vi "Destroy.vi"(11 "Data Value Reference in":refnum<data-value>) -> ()   [LabVIEW 2021, in "d20.lvlib" / "Node.lvclass"]
uses:
  Node.lvclass
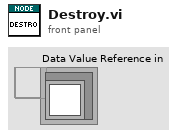
[diagram p1: front panel]
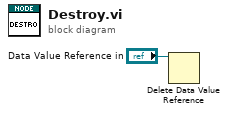
[diagram p0: block diagram]
diagram:
  n1 = Delete Data Value Reference(data value reference="Data Value Reference in") -> ()  [unwired: 1 in, 2 out]
